vi "Set Quiet Errors.vi"(9 "Quiet Errors?":bool=TRUE, 11 "Wavelength Meter.lvclass In":refnum<class "Wavelength Meter.lvclass">) -> (3 "Wavelength Meter.lvclass Out":refnum<class "Wavelength Meter.lvclass">)   [LabVIEW 2023, in "Wavelength Meter.lvclass"]
uses:
  Wavelength Meter.lvclass
  Wavelength Meter.lvclass/Wavelength Meter.ctl
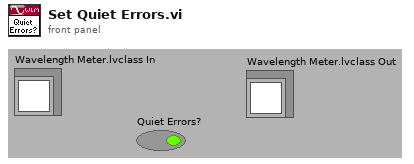
[diagram p1: front panel]
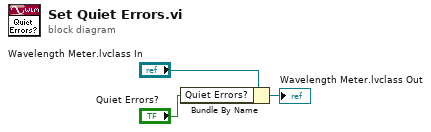
[diagram p0: block diagram]
diagram:
  n1 = Bundle By Name(cluster="Wavelength Meter.lvclass In", "Quiet Errors?"="Quiet Errors?") -> (→"Wavelength Meter.lvclass Out":refnum<class "Wavelength Meter.lvclass">)
